vi "Global 1.vi"() -> ()   [LabVIEW 2018]
panel:
  out "Maximum tentatives":dbl
  out "Code test":dbl
  out "Code secret":dbl
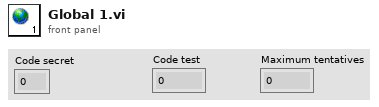
[diagram p1: front panel]
diagram:
